vi "Dashboard Main.vi"() -> ()   [LabVIEW 2014]
uses:
  <vilib>/event_ctls.llb/eventvkey.ctl
  <vilib>/Rock Robotics/WPI/Dashboard/WPI_DashboardLogging Global.vi
  <vilib>/Utility/config.llb/Write Key (String).vi
  <vilib>/Utility/config.llb/Write Key (I32).vi
  <vilib>/Utility/config.llb/NI_LVConfig.lvlib
  Custom/BB_AutonomousSelector.lvlib
panel:
  in  "Rec Mode":enum32{"Stop", "Record", "Playback"}(radio)
  in  "Vision":u16(ring) items=["Camera Off", "USB Camera", "IP Camera"]
  out "Camera IP":string
  out "Image Message":string="Timeout in Camera Communications"
  in  "Dashboard Tab":T1(tab)
  in  "Autonomous\nMode":u16(ring) items=["Mars Rock", "BETA_1BALL_STRAIGHT", "BETA_1BALL_CENTER_R", "BETA_2BALL_CENTER_R", "BETA_2BALL_CENTER_L"]
  out "Battery":dbl(slide) scale=11.0..13.0
  in  "Camera Settings":T2={"Frame Rate"=30, "Compression"=30, "Size"=1} {"Frame Rate" scale=1.0..30.0; "Size" items=["640x480", "320x240", "160x120"]}
  out "Mode":T3(ring)=enum."Auto Disabled"
  in  "DB Camera Config":bool
  out "fps":dbl format="%#.1g"
  out "Mbps":dbl format="%#.1g"
  out "Mbps 2":bool
  out "Air Pressure":dbl(knob) scale=0.0..130.0
  in  "DB/String 9":string
  in  "DB/String 8":string
  in  "DB/String 7":string
  in  "DB/String 6":string
  in  "DB/String 5":string
  in  "DB/String 4":string
  in  "DB/String 3":string
  in  "DB/String 2":string
  in  "DB/String 1":string
  in  "DB/String 0":string
  in  "DB/Slider 0":dbl(slide) scale=0.0..5.0
  in  "DB/Slider 1":dbl(slide) scale=0.0..5.0
  in  "DB/Slider 2":dbl(slide) scale=0.0..5.0
  in  "DB/Slider 3":dbl(slide) scale=0.0..5.0
  out "DB/LED 3":bool
  out "DB/LED 2":bool
  out "DB/LED 1":bool
  out "DB/LED 0":bool
  in  "DB/Button 3":bool
  in  "DB/Button 2":bool
  in  "DB/Button 1":bool
  in  "DB/Button 0":bool
  in  "Test Slider":dbl(slide) scale=0.0..100.0 scale format="%#_3g"
  in  "On/Off":bool caption="Solenoid"
  in  "Test Name":u16(ring) items=["Select the test to run...", "Example Test", "-------------------------------", "List of tests is built in robot code.", "Replace with your own automated tests."]
  in  "Test Tree":string(tree)
  in  "Motor":cluster{"Value":dbl, "Enable":bool} {"Value" scale=-1.0..1.0 scale format="%#_3g"}
  out "Progress":T4 {"Test Progress" scale=0.0..100.0}
  in  "Rev/Fwd":cluster{"Forward":bool, "Reverse":bool}
  in  "Test Ring":u16(ring) items=["Auto", "Fixed indoor", "Fixed outdoor 1", "Fixed outdoor 2", "Fixed fluorescent 1", "Fixed fluorescent 2", "Hold current"]
  in  "Listbox":i32(listbox)
  out "Tree":string(tree)
  out "Camera Image":T5(plugin-control)
  out "Boolean":bool
  # "This tab is a great place for autonomous settings and robot-specific values.\nPlacie controls and indicators inside this tab and match name to\nDashboard Variables on robot. You can also delete this comment."
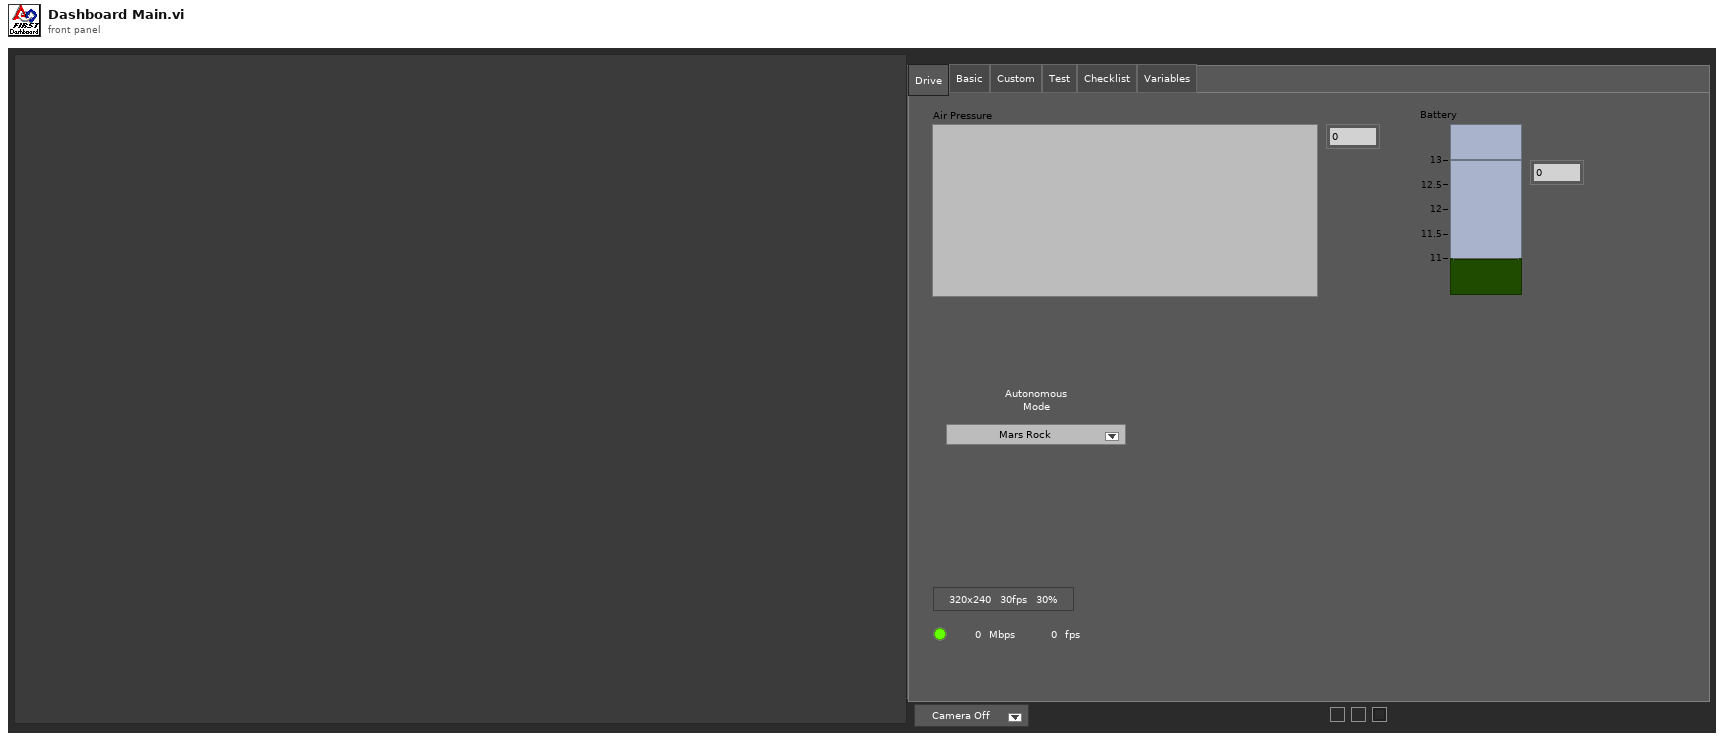
[diagram p1: front panel]
types:
  T1 = enum32{"Drive", "Basic", "Custom", "Test", "Checklist", "Variables"}
  T2 = cluster{"Frame Rate":i32, "Compression":i32, "Size":u16}
  T3 = enum8{"Tele-Op Disabled", "Tele-Op Enabled", "Auto Disabled", "Auto Enabled", "Test Disabled", "Test Enabled", ""}
  T4 = cluster{"Test Progress":u8, "Test Progress Text":string}
  T5 = typedef "IMAQ Image.ctl" = refnum<image>
  T6 = typedef "Image Type" = u32
  T7 = cluster{"Camera Image":refnum<vi>, "Dashboard Tab":refnum<vi>, "Boolean":refnum<vi>, "Vision":refnum<vi>, "Test Slider":refnum<vi>, "On/Off ":refnum<vi>, "Test Ring":refnum<vi>, "Rev/Fwd":refnum<vi>, "Rec Mode":refnum<vi>}
  T8 = cluster{"Digital Inputs":bool[], "Digital Outputs":bool[]}
  T9 = cluster{"Competition mode":bool, "Robot Link":bool, "Autonomous":bool, "Enabled":bool, "E-Stop":bool, "Simulated":bool, "TestMode":bool, "Docked Window":bool}
  T10 = typedef "NI_LVConfig.lvlib/Config Data RefNum.ctl" = refnum<k1>
  T11 = typedef "eventvkey.ctl" = enum16{"ASCII", "Enter", "Return", "Shift", "Ctrl", "Alt", "Cmd", "Opt", "Caps", "NumLock", "Clear", "Break", "Up", "Down", "Left", "Right", "Insert", "Delete", "Home", "End", "PageUp", "PageDown", "Escape", "Help", "Pause", "ScrollLock", "F1", "F2", "F3", "F4", "F5", "F6", "F7", "F8", "F9", "F10", "F11", "F12", "F13", "F14", "F15", "F16", "F17", "F18", "F19", "F20", "F21", "F22", "F23", "F24", "Play", "VolumeUp", "VolumeDown", "Mute", "Two Byte Char"}
  T12 = cluster{"Image Size":bool, "Image Type":bool, "Pixel Value":bool, "ROI Information":bool, "Zoom Factor":bool}
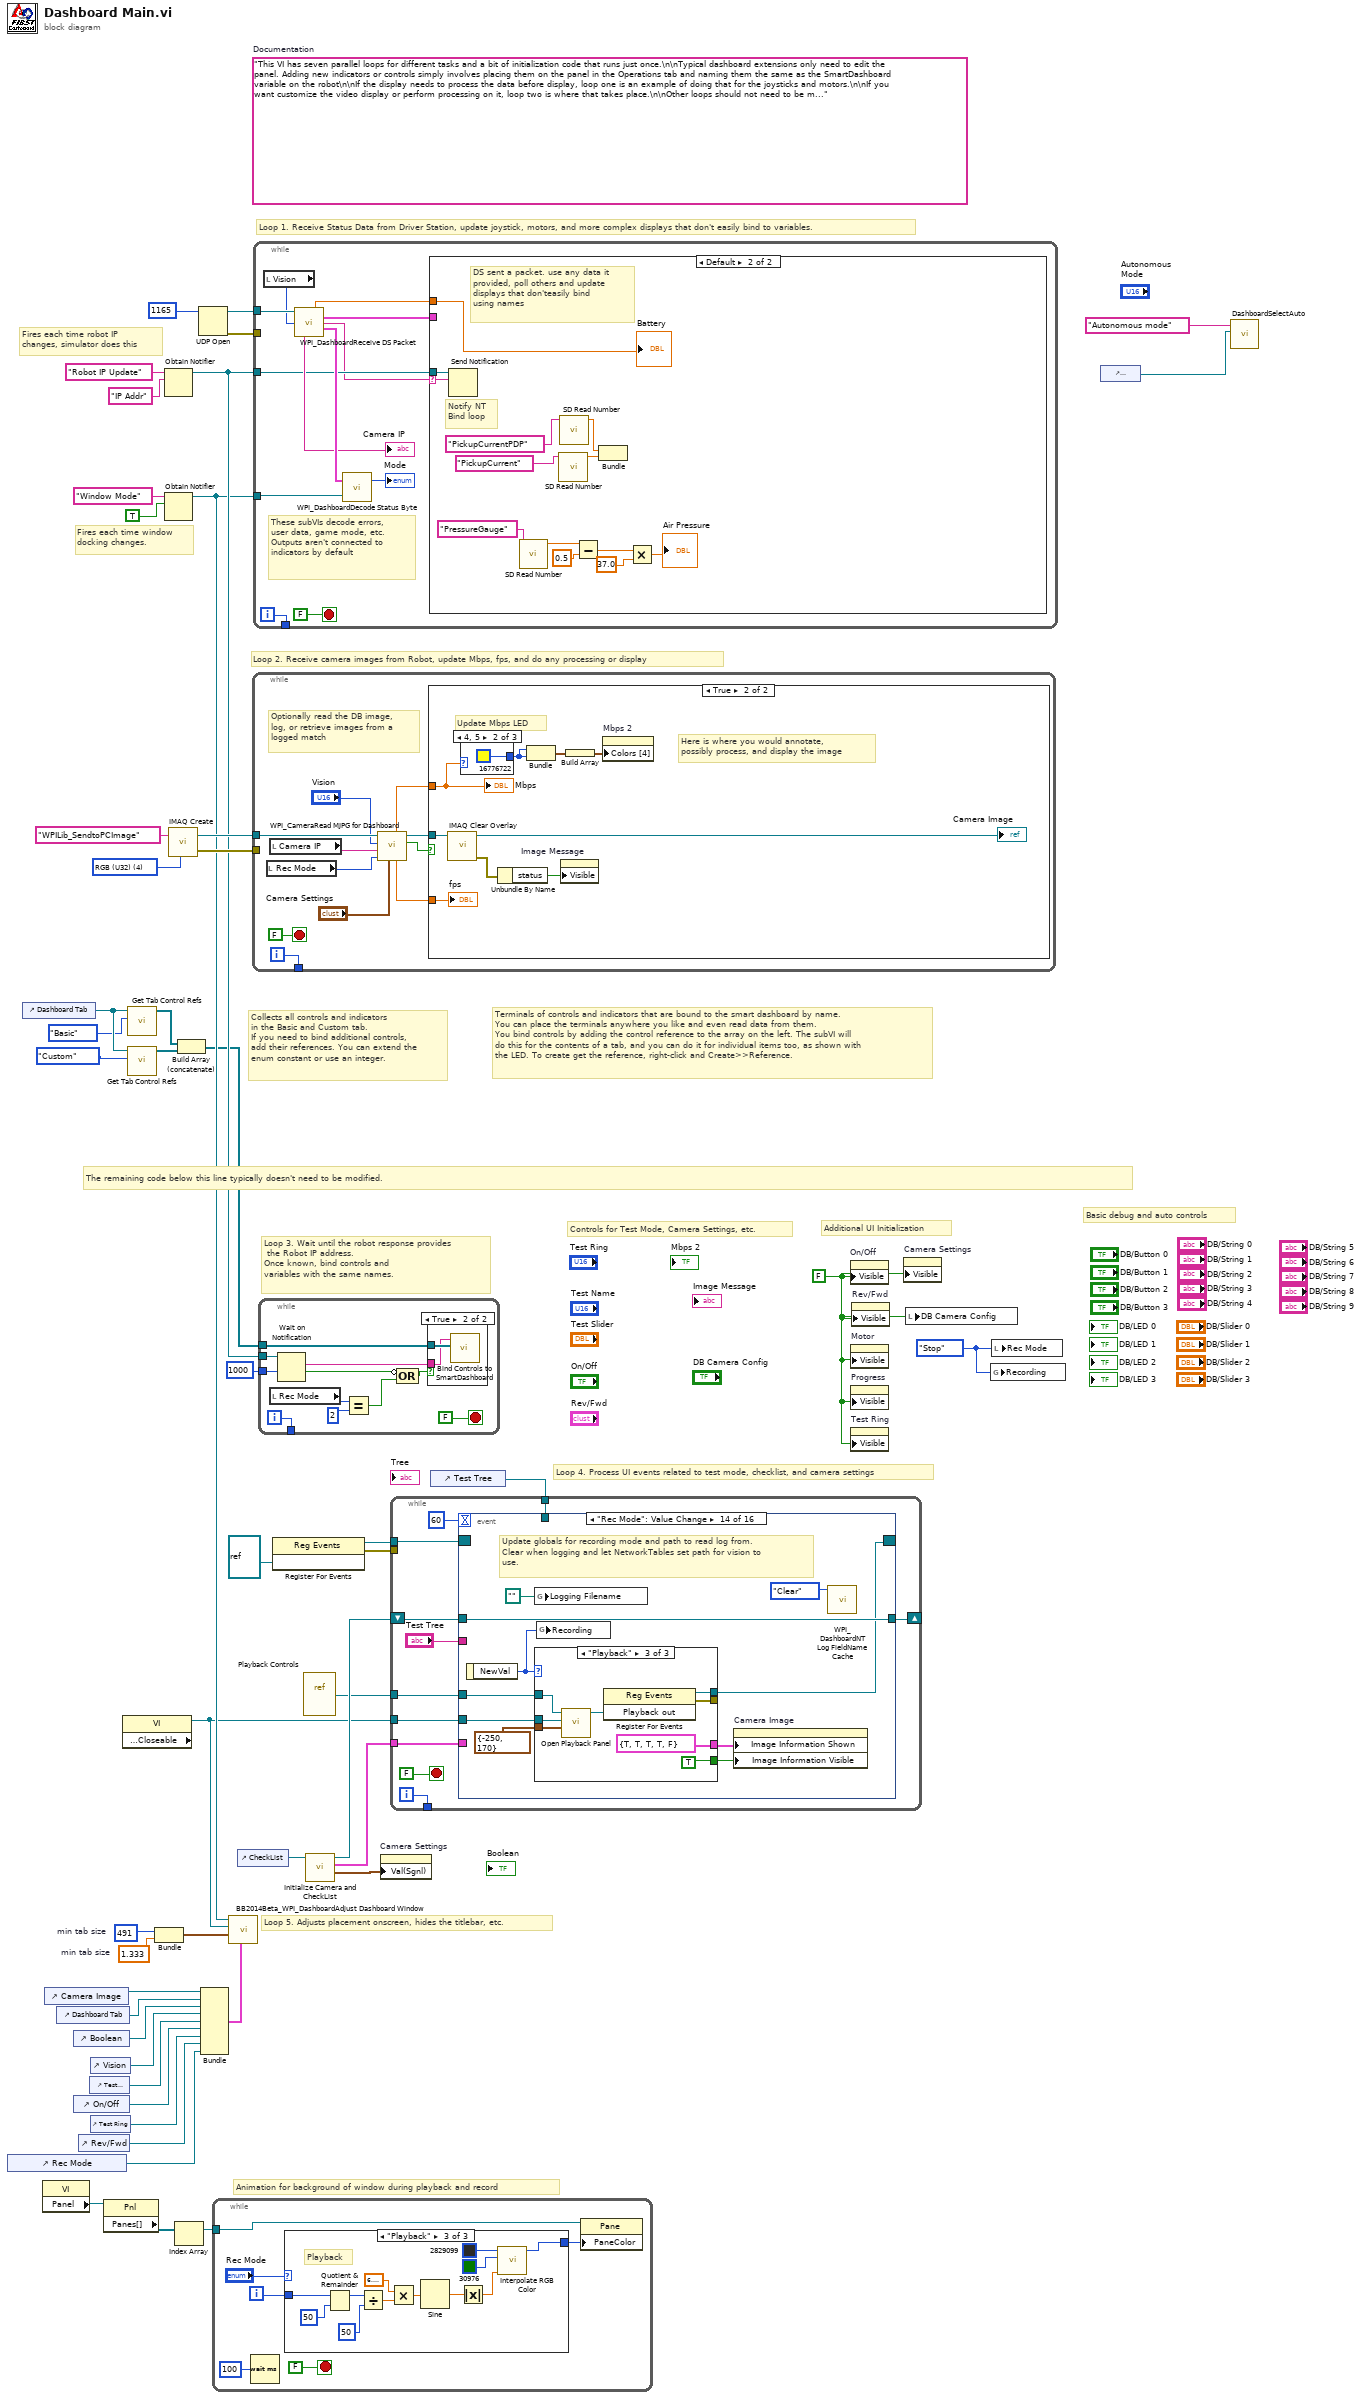
[diagram p0: block diagram]
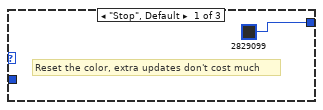
[diagram p2: hidden frame]
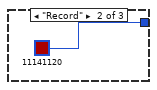
[diagram p3: hidden frame]
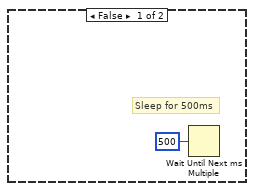
[diagram p5: hidden frame]
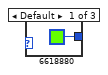
[diagram p6: hidden frame]
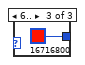
[diagram p7: hidden frame]
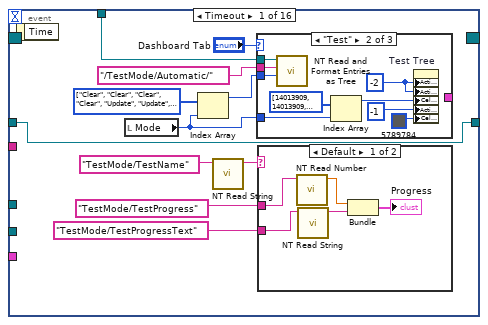
[diagram p8: hidden frame]
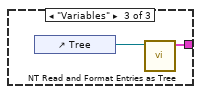
[diagram p10: hidden frame]
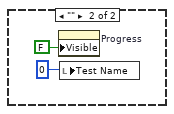
[diagram p11: hidden frame]
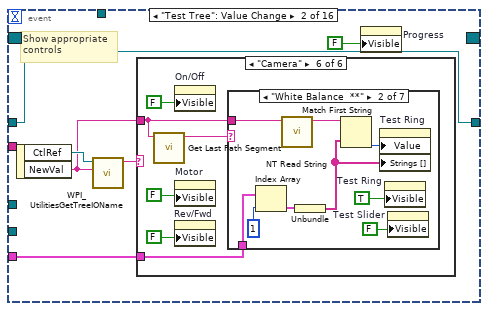
[diagram p12: hidden frame]
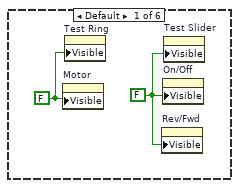
[diagram p13: hidden frame]
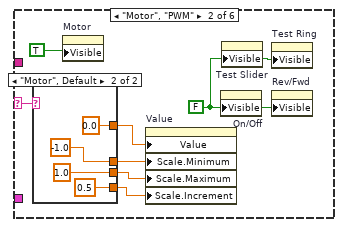
[diagram p14: hidden frame]
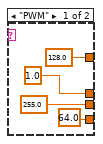
[diagram p15: hidden frame]
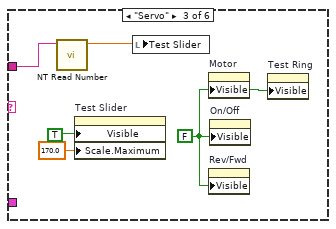
[diagram p16: hidden frame]
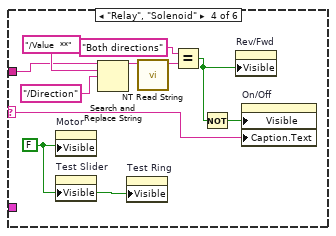
[diagram p17: hidden frame]
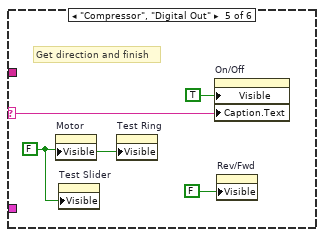
[diagram p18: hidden frame]
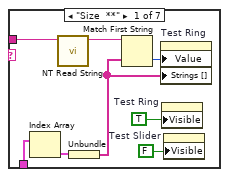
[diagram p19: hidden frame]
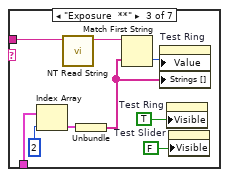
[diagram p20: hidden frame]
diagram:
  w10 = 491  # min tab size
  w9 = 1.333  # min tab size
  w24 = enum32{"Stop", "Record", "Playback"}."Stop" ("Rec Mode")
  w39 = FALSE ("Visible")
  (unwired) "This VI has seven parallel loops for different tasks and a bit of initialization code that runs just once.\n\nTypical dashboard extensions only need to edit the panel. Adding new indicators or controls simply involves placing them on the panel in the Operations tab and naming them the same as the SmartDashboard variable on the robot\n\nIf the display needs to process the data before display, loop one is an example of doing that for the joysticks and motors.\n\nIf you want customize the video display or perform processing on it, loop two is where that takes place.\n\nOther loops should not need to be modified. They are pretty standard, and document the task they perform."  # Documentation
  w48 = T6 4 items=["Grayscale (U8)", "Grayscale (I16)", "Grayscale (SGL)", "Complex (CSG)", "RGB (U32)", "HSL (U32)", "RGB (U64)"] ("Image Type")
  # "Basic debug and auto controls"
  # "Controls for Test Mode, Camera Settings, etc."
  # "Additional UI Initialization"
  # "Animation for background of window during playback and record"
  # "Fires each time robot IP\nchanges, simulator does this"
  # "Fires each time window\ndocking changes."
  # "Collects all controls and indicators\nin the Basic and Custom tab.\nIf you need to bind additional controls,\nadd their references. You can extend the\nenum constant or use an integer."
  # "The remaining code below this line typically doesn't need to be modified."
  # "Loop 4. Process UI events related to test mode, checklist, and camera settings"
  # "Terminals of controls and indicators that are bound to the smart dashboard by name.\nYou can place the terminals anywhere you like and even read data from them.\nYou bind controls by adding the control reference to the array on the left. The subVI will\ndo this for the contents of a tab, and you can do it for individual items too, as shown with\nthe LED. To create get the reference, right-click and Create>>Reference."
  # "Loop 3. Wait until the robot response provides\n the Robot IP address.\nOnce known, bind controls and\nvariables with the same names."
  # "Loop 5. Adjusts placement onscreen, hides the titlebar, etc."
  # "Loop 1. Receive Status Data from Driver Station, update joystick, motors, and more complex displays that don't easily bind to variables."
  # "Loop 2. Receive camera images from Robot, update Mbps, fps, and do any processing or display"
  n1 = control-ref of="Rec Mode"() -> (w11:refnum<vi>)
  n2 = control-ref of="Dashboard Tab"() -> (w22:refnum<vi>)
  n3 = property class="VI"() -> ("Panel"=w33:refnum<vi>)  [unwired: 2 in, 2 out]
  n4 = control-ref of="Camera Image"() -> (w18:refnum<vi>)
  n5 = control-ref of="Dashboard Tab"() -> (w17:refnum<vi>)
  n6 = control-ref of="Boolean"() -> (w7:refnum<vi>)
  n7 = control-ref of="On/Off"() -> (w14:refnum<vi>)
  n8 = control-ref of="Rev/Fwd"() -> (w12:refnum<vi>)
  n9 = control-ref of="Test Slider"() -> (w15:refnum<vi>)
  n10 = control-ref of="Vision"() -> (w16:refnum<vi>)
  n11 = control-ref of="Test Ring"() -> (w13:refnum<vi>)
  n12 = property class="Pnl"(reference=w33) -> ("Panes[]"=w34:refnum<vi>[])  [unwired: 1 in, 2 out]
  n13 = property class="VI" props=["Front Panel.Closeable"]() -> (reference out=w23:refnum<vi>)  [unwired: 2 in, 2 out]
  n14 = call <vilib>:"Get Tab Control Refs.vi"("Page Index"=T1."Basic" ("Dashboard Tab"), "TabControl in"=w22) -> ("ControlsOnPage"=w20:refnum<vi>[])  [unwired: 9 in]
  n15 = call <vilib>:"Get Tab Control Refs.vi"("Page Index"=T1."Custom" ("Dashboard Tab"), "TabControl in"=w22) -> ("ControlsOnPage"=w21:refnum<vi>[])  [unwired: 9 in]
  n16 = Bundle("min tab size"=w10, "min tab size"=w9) -> (w8:cluster{"min tab size":i32, "min tab size":dbl})  [unwired: 1 in]
  n17 = Obtain Notifier(name (unnamed)="Robot IP Update", notification data type="IP Addr" ("name (unnamed)")) -> (notifier out=w42:refnum<notifier>)  [unwired: 2 in, 2 out]
  n18 = Obtain Notifier(name (unnamed)="Window Mode", notification data type=TRUE) -> (notifier out=w26:refnum<notifier>)  [unwired: 2 in, 2 out]
  n19 = call "IMAQ Create"("Image Name"="WPILib_SendtoPCImage", "Image Type"=w48) -> ("New Image"=w46:T5, "error out"=w45:errorcluster)  [unwired: 2 in, 1 out]
  n20 = Index Array(array=w34) -> (element=w32:refnum<vi>)  [unwired: 1 in]
  n21 = Build Array (concatenate)(w20, w21) -> (w19:refnum<vi>[])
  n22 = UDP Open(11:u16 1165 ("port")) -> (port=w49:refnum<k16>, 0:w4:errorcluster)  [unwired: 2 in, 3 out]
  n23 = Bundle("Camera Image"=w18, "Dashboard Tab"=w17, "Boolean"=w7, "Vision"=w16, "Test Slider"=w15, "On/Off"=w14, "Test Ring"=w13, "Rev/Fwd"=w12, "Rec Mode"=w11) -> (w3:T7)  [unwired: 1 in]
  n24 = while {
    tunnel: w32 -> [w52]
    i -> [w55]
    stop <- FALSE stop-if-true
    n25 = Wait (ms)(milliseconds to wait=u32 100) -> ()  [unwired: 1 out]
    n26 = case shown="\"Playback\"" "Rec Mode" {
      tunnel: w55 -> [_ _ w70]
      tunnel: [u32 2829099 ("Base Color") u32 11141120 ("Target Color") w59] -> w51
      frame "Stop", Default {
        # "Reset the color, extra updates don't cost much"
      }
      frame "Record" {
      }
      frame "Playback" {
        # "Playback"
        n27 = Quotient & Remainder(x=w70, y=u32 50 ("milliseconds to wait")) -> (x-y*floor(x/y)=w66:u32)  [unwired: 1 out]
        n28 = Divide(x=w66, y=u32 50 ("milliseconds to wait")) -> (x/y=w63:dbl)
        n29 = Multiply(x=6.283185307179586, y=w63) -> (x*y=w68:dbl)
        n30 = Sine(x=w68) -> (sin(x)=w67:dbl)
        n31 = Absolute Value(x=w67) -> (abs(x)=w60:dbl)
        n32 = call "Interpolate RGB Color.vi"("Proportion"=w60, "Target Color"=u32 30976, "Base Color"=u32 2829099) -> ("Result Color"=w59:u32)  [unwired: 8 in]
      }
    }
    n33 = property class="Pane"(reference=w52, "PaneColor"=w51) -> ()  [unwired: 1 in, 2 out]
  }
  n34 = call "BB2014Beta_WPI_DashboardAdjust Dashboard Window.vi"("Sizing Refnums"=w3, "Size Constraints"=w8, "VI"=w23, "Notifier in"=w26) -> ()  [unwired: 8 in]
  n35 = control-ref of="CheckList"() -> (w25:refnum<vi>)
  n36 = while {
    tunnel: w46 -> [w79]
    tunnel: w45 -> [_]
    tunnel: [w80] -> _
    i -> [w80]
    stop <- FALSE stop-if-true
    # "Optionally read the DB image,\nlog, or retrieve images from a\nlogged match"
    n37 = local read "Rec Mode"() -> (w73:enum32{"Stop", "Record", "Playback"})
    n38 = local read "Camera IP"() -> (w71:string)
    n39 = call <vilib>:"WPI_CameraRead MJPG for Dashboard.vi"("Camera Settings"="Camera Settings", "Rec Mode"=w73, "Camera IP"=w71, "Vision"="Vision", "Refnum in"=w79) -> ("Active"=w77:bool, "Refnum out"=w78:T5, "FPS"=w76:dbl, "Bandwidth (Mbps)"=w75:dbl)  [unwired: 3 in]
    n40 = case shown="True" w77 {
      tunnel: w78 -> [_ w86]
      tunnel: w75 -> [_ w85]
      tunnel: w76 -> [_ w83]
      frame False {
        # "Sleep for 500ms"
        n41 = Wait Until Next ms Multiple(millisecond multiple=u32 500) -> ()  [unwired: 1 out]
      }
      frame True {
        # "Here is where you would annotate,\npossibly process, and display the image"
        # "Update Mbps LED"
        n42 = call "IMAQ Clear Overlay"("Image"=w86) -> ("error out"=w90:errorcluster, "Image Out"=→"Camera Image":T5)  [unwired: 2 in, 7 out]
        n43 = case shown="4, 5" w85 {
          tunnel: [u32 6618880 ("Color Box") u32 16776722 ("Color Box") u32 16716800 ("Color Box")] -> w87
          frame Default {
          }
          frame 4, 5 {
          }
          frame 6.. {
          }
        }
        n44 = Unbundle By Name(w90) -> ("status"=w91:bool)
        n45 = Bundle("Color Box"=w87, "Color Box"=w87) -> (w89:cluster{"Color Box":u32, "Color Box":u32})  [unwired: 1 out]
        n46 = property on="Image Message" class="Str"("Visible"=w91) -> ()  [unwired: 2 in, 2 out]
        n47 = Build Array(w89) -> (w88:cluster{"Color Box":u32, "Color Box":u32}[])
        n48 = property on="Mbps 2" class="Bool (strict)"("Colors [4]"=w88) -> ()  [unwired: 2 in, 2 out]
        "Mbps" <- w85
        "fps" <- w83
      }
    }
  }
  n49 = while {
    tunnel: w49 -> [w104]
    tunnel: w42 -> [w99]
    tunnel: w26 -> [w103]
    tunnel: [w100] -> _
    tunnel: w4 -> [_]
    i -> [w100]
    stop <- FALSE stop-if-true
    # "These subVIs decode errors, user data, game mode, etc.\nOutputs aren't connected to indicators by default"
    n50 = local read "Vision"() -> (w95:u16)
    n51 = call <vilib>:"WPI_DashboardReceive DS Packet.vi"("Recv Socket"=w104, "Vision"=w95) -> ("Battery"=w97:sgl, "Driver Station"=w98:T8, "Robot IP Address"=w96:string, "Status"=w105:T9, "Camera IP Address"=→"Camera IP":string)  [unwired: 1 in, 8 out]
    n52 = call <vilib>:"WPI_DashboardDecode Status Byte.vi"("Window Mode Notifier"=w103, "Status"=w105) -> ("Mode"=→"Mode":T3)  [unwired: 1 out]
    n53 = case shown="Default" w96 {
      selector: w96 -> [_ w118]
      tunnel: w99 -> [_ w119]
      tunnel: w98 -> [_ _]
      tunnel: w97 -> [_ w107]
      frame "0.0.0.0" {
        # "DS not sending packets, or no robot exists yet.\nDon't poll the variables"
      }
      frame Default {
        # "Notify NT\nBind loop"
        # "DS sent a packet. use any data it\nprovided, poll others and update\ndisplays that don'teasily bind\nusing names"
        n54 = Send Notification(notification=w118, notifier=w119) -> ()  [unwired: 1 in, 2 out]
        n55 = call <vilib>:"SD Read Number.vi"("Name"="PressureGauge") -> ("Numeric"=w116:dbl)  [unwired: 8 in, 2 out]
        n56 = call <vilib>:"SD Read Number.vi"("Name"="PickupCurrent") -> ("Numeric"=w110:dbl)  [unwired: 8 in, 2 out]
        n57 = call <vilib>:"SD Read Number.vi"("Name"="PickupCurrentPDP") -> ("Numeric"=w108:dbl)  [unwired: 8 in, 2 out]
        n58 = Subtract(x=w116, y=0.5) -> (x-y=w114:dbl)
        n59 = Bundle("Numeric"=w108, "Numeric"=w110) -> ()  [unwired: 1 in, 1 out]
        n60 = Multiply(x=w114, y=37.0) -> (x*y=→"Air Pressure":dbl)
        "Battery" <- w107
      }
    }
  }
  n61 = while {
    tunnel: w19 -> [w130]
    tunnel: w42 -> [w128]
    tunnel: [w126] -> _
    tunnel: u32 1000 ("milliseconds to wait") -> [w125]
    i -> [w126]
    stop <- FALSE stop-if-true
    n62 = local read "Rec Mode"() -> (w121:enum32{"Stop", "Record", "Playback"})
    n63 = Wait on Notification(notifier=w128, timeout in ms (-1)=w125) -> (notification=w127:string, timed out?=w123:bool)  [unwired: 2 in, 2 out]
    n64 = Equal?(x=w121, y=u16 2 ("Rec Mode")) -> (x = y?=w122:bool)
    n65 = Compound Arithmetic op=OR(invert w123, w122) -> (w124:bool)
    n66 = case shown="True" w124 {
      tunnel: w130 -> [_ w132]
      tunnel: w127 -> [_ w131]
      frame False {
      }
      frame True {
        n67 = call <vilib>:"Bind Controls to SmartDashboard.vi"("Bound Control Refs"=w132, "Server IP Address"=w131) -> ()  [unwired: 10 in]
      }
    }
  }
  n68 = register-events(refnum<vi> refnum) -> (reference out=w30:refnum<event-registration>, error out=w29:errorcluster)  [unwired: 2 in]
  n69 = vi-ref "Playback Controls.vi"() -> (w31:refnum<vi>)
  n70 = call "Initialize Camera and CheckList.vi"("ListBox in"=w25) -> ("Cluster"=w37:cluster{"value":i32, "value":i32, "index":i32}, "Array"=w38:cluster{string[]}[], "File Refnum"=w36:T10)  [unwired: 8 in]
  n71 = property on="Camera Settings" class="Clust (strict)"("Val(Sgnl)"=w37) -> ()  [unwired: 2 in, 2 out]
  n72 = control-ref of="Test Tree"() -> (w35:refnum<vi>)
  n73 = while {
    tunnel: w38 -> [w140]
    shift-right: [w139] -> _
    shift-left: w36 -> [w138]
    tunnel: [w137] -> _
    tunnel: w35 -> [w136]
    tunnel: w31 -> [w135]
    tunnel: w30 -> [w134]
    tunnel: w29 -> [_]
    tunnel: w23 -> [w133]
    i -> [w137]
    stop <- FALSE stop-if-true
    n74 = event shown="[13] \"Rec Mode\": Value Change" {
      selector: w134 -> [_ _ _ _ _ _ _ _ _ _ _ _ _ _ _ _]
      dyn-events: [_ _ _ _ _ _ _ _ _ _ _ _ _ w378 _ _] -> _
      timeout: u32 60 ("milliseconds to wait") -> [_ _ _ _ _ _ _ _ _ _ _ _ _ _ _ _]
      tunnel: w136 -> [w150 _ _ _ _ _ _ _ _ _ _ _ _ _ _ _]
      tunnel: "Test Tree" -> [_ _ _ _ _ _ _ _ w347 w355 w357 w361 w369 _ _ _]
      tunnel: w140 -> [_ w174 _ _ _ _ w311 w341 _ _ _ _ _ _ _ _]
      tunnel: [w144 w173 w272 w277 w285 w297 w310 w334 w346 w353 w356 w360 w368 w380 w394 w395] -> w139
      tunnel: w138 -> [w144 w173 w272 w277 w285 w297 w309 w334 w346 w353 w356 w360 w368 w380 w394 w395]
      tunnel: w135 -> [_ _ _ _ _ _ _ _ _ _ _ _ _ w381 _ w398]
      tunnel: w133 -> [_ _ _ _ _ _ _ _ _ _ _ _ _ w376 _ _]
      event Timeout {
        w149 = enum16{"Update", "Clear"}[] [enum."Clear", enum."Clear", enum."Clear", enum."Clear", enum."Update", enum."Update", enum."Clear"] items=["Update", "Clear"]
        n75 = event-data() -> ()  [unwired: 1 in, 1 out]
        n76 = local read "Mode"() -> (w147:T3)
        n77 = Index Array(array=w149, index=w147) -> (element=w148:enum16{"Update", "Clear"})
        n78 = call <vilib>:"NT Read String.vi"("Name"="TestMode/TestName") -> ("String"=w153:string)  [unwired: 9 in, 1 out]
        n79 = case shown="\"Test\"" "Dashboard Tab" {
          tunnel: w150 -> [_ w163 _]
          tunnel: "/TestMode/Automatic/" ("Name Pattern") -> [_ w162 _]
          tunnel: w148 -> [_ w161 _]
          tunnel: w147 -> [_ w159 _]
          tunnel: [_ _ w165] -> _
          frame "Custom", Default {
          }
          frame "Test" {
            w158 = -2 ("Active Item:Row Number")
            n80 = call <vilib>:"NT Read and Format Entries as Tree.vi"("Operation"=w161, "Name Pattern"=w162, "Tree Refnum"=w163) -> ()  [unwired: 7 in, 2 out]
            n81 = Index Array(array=u32[] [14013909, 14013909, 14013909, 14013909, 14013909, 16777215, 14013909], index=w159) -> (element=w157:u32)
            n82 = property on="Test Tree" class="Tree (strict)"("Active Item Row Number"=w158, "ActiveColNum"=w158, "CellBG"=w157, "Active Item Row Number"=-1 ("Active Item:Row Number"), "CellBG"=u32 5789784 ("Color Box")) -> ()  [unwired: 2 in, 2 out]
          }
          frame "Variables" {
            n83 = control-ref of="Tree"() -> (w164:refnum<vi>)
            n84 = call <vilib>:"NT Read and Format Entries as Tree.vi"("Tree Refnum"=w164) -> ("Formatted Strings"=w165:cluster{"Name":string, "Value":string}[])  [unwired: 9 in, 1 out]
          }
        }
        n85 = case shown="Default" w153 {
          tunnel: "TestMode/TestProgress" ("Name") -> [w167 _]
          tunnel: "TestMode/TestProgressText" ("Name") -> [w166 _]
          frame Default {
            n86 = call <vilib>:"NT Read Number.vi"("Name"=w167) -> ("Numeric"=w168:dbl)  [unwired: 9 in, 1 out]
            n87 = call <vilib>:"NT Read String.vi"("Name"=w166) -> ("String"=w169:string)  [unwired: 9 in, 1 out]
            n88 = Bundle("Numeric"=w168, "String"=w169) -> (→"Progress":cluster{"Numeric":dbl, "String":string})  [unwired: 1 in]
          }
          frame "" {
            n89 = property on="Progress" class="Clust (strict)"("Visible"=FALSE) -> ()  [unwired: 2 in, 2 out]
            n90 = local write "Test Name"(u16 0) -> ()
          }
        }
      }
      event "Test Tree": Value Change {
        # "Show appropriate\ncontrols"
        n91 = event-data() -> ("CtlRef"=w177:refnum<vi>, "NewVal"=w175:string)  [unwired: 1 in]
        n92 = call <vilib>:"WPI_UtilitiesGetTreeIOName.vi"("NewVal"=w175, "TreeControl in"=w177) -> ("I/O Name"=w178:string)  [unwired: 9 in]
        n93 = case shown="\"Camera\"" w178 {
          selector: w178 -> [_ w185 _ w203 w212 _]
          tunnel: w175 -> [_ _ w200 w202 _ w219]
          tunnel: w174 -> [_ _ _ _ _ w218]
          frame Default {
            w180 = FALSE ("Visible")
            w179 = FALSE ("Visible")
            n94 = property on="Motor" class="Clust (strict)"("Visible"=w179) -> ()  [unwired: 2 in, 2 out]
            n95 = property on="Test Ring" class="Ring (strict)"("Visible"=w179) -> ()  [unwired: 2 in, 2 out]
            n96 = property on="Rev/Fwd" class="Clust (strict)"("Visible"=w180) -> ()  [unwired: 2 in, 2 out]
            n97 = property on="On/Off" class="Bool (strict)"("Visible"=w180) -> ()  [unwired: 2 in, 2 out]
            n98 = property on="Test Slider" class="Slide (strict)"("Visible"=w180) -> ()  [unwired: 2 in, 2 out]
          }
          frame "Motor", "PWM" {
            w186 = FALSE ("Visible")
            n99 = case shown="\"Motor\", Default" w185 {
              tunnel: [1.0 ("Value") -1.0 ("Value")] -> w184
              tunnel: [255.0 ("Value") 1.0 ("Value")] -> w183
              tunnel: [128.0 ("Value") 0.0 ("Value")] -> w182
              tunnel: [64.0 ("Value") 0.5 ("Value")] -> w181
              frame "PWM" {
              }
              frame "Motor", Default {
              }
            }
            n100 = property on="Motor" class="Clust (strict)"("Visible"=TRUE) -> ()  [unwired: 2 in, 2 out]
            n101 = property on="Value" class="Slide (strict)"("Value"=w182, "Scale.Minimum"=w184, "Scale.Maximum"=w183, "Scale.Increment"=w181) -> ()  [unwired: 2 in, 2 out]
            n102 = property on="On/Off" class="Bool (strict)"("Visible"=w186) -> ()  [unwired: 2 in, 2 out]
            n103 = property on="Test Slider" class="Slide (strict)"("Visible"=w186) -> ()  [unwired: 2 in, 2 out]
            n104 = property on="Test Ring" class="Ring (strict)"("Visible"=w186) -> ()  [unwired: 2 in, 2 out]
            n105 = property on="Rev/Fwd" class="Clust (strict)"("Visible"=w186) -> ()  [unwired: 2 in, 2 out]
          }
          frame "Servo" {
            w198 = FALSE ("Visible")
            n106 = call <vilib>:"NT Read Number.vi"("Name"=w200) -> ("Numeric"=w199:dbl)  [unwired: 9 in, 1 out]
            n107 = property on="Test Slider" class="Slide (strict)"("Visible"=TRUE, "Scale.Maximum"=170.0 ("Scale.Range:Maximum")) -> ()  [unwired: 2 in, 2 out]
            n108 = local write "Test Slider"(w199) -> ()
            n109 = property on="Motor" class="Clust (strict)"("Visible"=w198) -> ()  [unwired: 2 in, 2 out]
            n110 = property on="Rev/Fwd" class="Clust (strict)"("Visible"=w198) -> ()  [unwired: 2 in, 2 out]
            n111 = property on="On/Off" class="Bool (strict)"("Visible"=w198) -> ()  [unwired: 2 in, 2 out]
            n112 = property on="Test Ring" class="Ring (strict)"("Visible"=w198) -> ()  [unwired: 2 in, 2 out]
          }
          frame "Relay", "Solenoid" {
            w201 = FALSE ("Visible")
            n113 = property on="Motor" class="Clust (strict)"("Visible"=w201) -> ()  [unwired: 2 in, 2 out]
            n114 = property on="Test Slider" class="Slide (strict)"("Visible"=w201) -> ()  [unwired: 2 in, 2 out]
            n115 = Search and Replace String(input string=w202, search string="/Value  **", replace string="/Direction") -> (result string=w208:string)  [unwired: 5 in, 3 out]
            n116 = property on="Test Ring" class="Ring (strict)"("Visible"=w201) -> ()  [unwired: 2 in, 2 out]
            n117 = call <vilib>:"NT Read String.vi"("Name"=w208) -> ("String"=w206:string)  [unwired: 9 in, 1 out]
            n118 = Equal?(x="Both directions", y=w206) -> (x = y?=w204:bool)
            n119 = Not(x=w204) -> (.not. x?=w205:bool)
            n120 = property on="Rev/Fwd" class="Clust (strict)"("Visible"=w204) -> ()  [unwired: 2 in, 2 out]
            n121 = property on="On/Off" class="Bool (strict)"("Visible"=w205, "Caption.Text"=w203) -> ()  [unwired: 2 in, 2 out]
          }
          frame "Compressor", "Digital Out" {
            w211 = FALSE ("Visible")
            # "Get direction and finish"
            n122 = property on="Motor" class="Clust (strict)"("Visible"=w211) -> ()  [unwired: 2 in, 2 out]
            n123 = property on="Test Slider" class="Slide (strict)"("Visible"=w211) -> ()  [unwired: 2 in, 2 out]
            n124 = property on="Test Ring" class="Ring (strict)"("Visible"=w211) -> ()  [unwired: 2 in, 2 out]
            n125 = property on="On/Off" class="Bool (strict)"("Visible"=TRUE, "Caption.Text"=w212) -> ()  [unwired: 2 in, 2 out]
            n126 = property on="Rev/Fwd" class="Clust (strict)"("Visible"=FALSE) -> ()  [unwired: 2 in, 2 out]
          }
          frame "Camera" {
            n127 = call <vilib>:"Get Last Path Segment.vi"("String in"=w219) -> ("String out"=w220:string)  [unwired: 10 in]
            n128 = property on="On/Off" class="Bool (strict)"("Visible"=FALSE) -> ()  [unwired: 2 in, 2 out]
            n129 = property on="Motor" class="Clust (strict)"("Visible"=FALSE) -> ()  [unwired: 2 in, 2 out]
            n130 = property on="Rev/Fwd" class="Clust (strict)"("Visible"=FALSE) -> ()  [unwired: 2 in, 2 out]
            n131 = case shown="\"White Balance  **\"" w220 {
              tunnel: w219 -> [w226 w235 w244 w253 w262 _ w268]
              tunnel: w218 -> [w224 w232 w241 w250 w259 _ _]
              frame "Size  **" {
                n132 = Index Array(array=w224) -> (element=w223:cluster{string[]})  [unwired: 1 in]
                n133 = call <vilib>:"NT Read String.vi"("Name"=w226) -> ("String"=w225:string)  [unwired: 9 in, 1 out]
                n134 = Unbundle(w223) -> (w221:string[])
                n135 = Match First String(2:w221, 3:w225) -> (0:w222:i32)  [unwired: 1 out]
                n136 = property on="Test Ring" class="Ring (strict)"("Value"=w222, "Strings []"=w221) -> ()  [unwired: 2 in, 2 out]
                n137 = property on="Test Ring" class="Ring (strict)"("Visible"=TRUE) -> ()  [unwired: 2 in, 2 out]
                n138 = property on="Test Slider" class="Slide (strict)"("Visible"=FALSE) -> ()  [unwired: 2 in, 2 out]
              }
              frame "White Balance  **" {
                n139 = Index Array(array=w232, index=1) -> (element=w233:cluster{string[]})
                n140 = call <vilib>:"NT Read String.vi"("Name"=w235) -> ("String"=w234:string)  [unwired: 9 in, 1 out]
                n141 = Unbundle(w233) -> (w230:string[])
                n142 = Match First String(2:w230, 3:w234) -> (0:w229:i32)  [unwired: 1 out]
                n143 = property on="Test Ring" class="Ring (strict)"("Value"=w229, "Strings []"=w230) -> ()  [unwired: 2 in, 2 out]
                n144 = property on="Test Ring" class="Ring (strict)"("Visible"=TRUE) -> ()  [unwired: 2 in, 2 out]
                n145 = property on="Test Slider" class="Slide (strict)"("Visible"=FALSE) -> ()  [unwired: 2 in, 2 out]
              }
              frame "Exposure  **" {
                n146 = Index Array(array=w241, index=2) -> (element=w242:cluster{string[]})
                n147 = call <vilib>:"NT Read String.vi"("Name"=w244) -> ("String"=w243:string)  [unwired: 9 in, 1 out]
                n148 = Unbundle(w242) -> (w238:string[])
                n149 = Match First String(2:w238, 3:w243) -> (0:w239:i32)  [unwired: 1 out]
                n150 = property on="Test Ring" class="Ring (strict)"("Value"=w239, "Strings []"=w238) -> ()  [unwired: 2 in, 2 out]
                n151 = property on="Test Ring" class="Ring (strict)"("Visible"=TRUE) -> ()  [unwired: 2 in, 2 out]
                n152 = property on="Test Slider" class="Slide (strict)"("Visible"=FALSE) -> ()  [unwired: 2 in, 2 out]
              }
              frame "Exposure Priority  **" {
                n153 = Index Array(array=w250, index=3) -> (element=w251:cluster{string[]})
                n154 = call <vilib>:"NT Read String.vi"("Name"=w253) -> ("String"=w252:string)  [unwired: 9 in, 1 out]
                n155 = Unbundle(w251) -> (w247:string[])
                n156 = Match First String(2:w247, 3:w252) -> (0:w248:i32)  [unwired: 1 out]
                n157 = property on="Test Ring" class="Ring (strict)"("Value"=w248, "Strings []"=w247) -> ()  [unwired: 2 in, 2 out]
                n158 = property on="Test Ring" class="Ring (strict)"("Visible"=TRUE) -> ()  [unwired: 2 in, 2 out]
                n159 = property on="Test Slider" class="Slide (strict)"("Visible"=FALSE) -> ()  [unwired: 2 in, 2 out]
              }
              frame "Color Enable  **" {
                n160 = Index Array(array=w259, index=4) -> (element=w260:cluster{string[]})
                n161 = call <vilib>:"NT Read String.vi"("Name"=w262) -> ("String"=w261:string)  [unwired: 9 in, 1 out]
                n162 = Unbundle(w260) -> (w256:string[])
                n163 = Match First String(2:w256, 3:w261) -> (0:w257:i32)  [unwired: 1 out]
                n164 = property on="Test Ring" class="Ring (strict)"("Value"=w257, "Strings []"=w256) -> ()  [unwired: 2 in, 2 out]
                n165 = property on="Test Ring" class="Ring (strict)"("Visible"=TRUE) -> ()  [unwired: 2 in, 2 out]
                n166 = property on="Test Slider" class="Slide (strict)"("Visible"=FALSE) -> ()  [unwired: 2 in, 2 out]
              }
              frame Default {
                n167 = property on="Test Ring" class="Ring (strict)"("Visible"=FALSE) -> ()  [unwired: 2 in, 2 out]
                n168 = property on="Test Slider" class="Slide (strict)"("Visible"=FALSE) -> ()  [unwired: 2 in, 2 out]
              }
              frame "Brightness  **", "Color Level  **", "Compression  **", "FPS  **", "Sharpness  **" {
                n169 = call <vilib>:"NT Read Number.vi"("Name"=w268) -> ("Numeric"=w267:dbl)  [unwired: 9 in, 1 out]
                n170 = local write "Test Slider"(w267) -> ()
                n171 = property on="Test Slider" class="Slide (strict)"("Visible"=TRUE, "Scale.Maximum"=100.0 ("Scale.Range:Maximum")) -> ()  [unwired: 2 in, 2 out]
                n172 = property on="Test Ring" class="Ring (strict)"("Visible"=FALSE) -> ()  [unwired: 2 in, 2 out]
              }
            }
          }
        }
        n173 = property on="Progress" class="Clust (strict)"("Visible"=FALSE) -> ()  [unwired: 2 in, 2 out]
      }
      event "Test Name": Mouse Enter {
        # "Populate the ring with the list of tests"
        n174 = event-data() -> ()  [unwired: 1 in, 1 out]
        n175 = call <vilib>:"NT Read String Array.vi"("Name"="TestMode/TestList") -> ("String Array"=w276:string[])  [unwired: 9 in, 1 out]
        n176 = Build Array (concatenate)("Select the test to run...", w276) -> (w275:string[])
        n177 = property on="Test Name" class="Ring (strict)"("Strings []"=w275) -> ()  [unwired: 2 in, 2 out]
      }
      event "Test Name": Value Change {
        w278 = FALSE ("Visible")
        # "Tell the robot the test name to run"
        n178 = event-data() -> ("NewVal"=w282:u16)  [unwired: 1 in]
        n179 = property on="Test Name" class="Ring (strict)"() -> ("Strings []"=w283:string[])  [unwired: 2 in, 2 out]
        n180 = local write "Progress"(T4 {"Test Progress"=0, "Test Progress Text"=""} ("Progress")) -> ()
        n181 = Index Array(array=w283, index=w282) -> (element=w281:string)
        n182 = call <vilib>:"NT Write String.vi"("String"=w281, "Name"="TestMode/TestName") -> ()  [unwired: 9 in, 1 out]
        n183 = property on="Progress" class="Clust (strict)"("Visible"=TRUE) -> ()  [unwired: 2 in, 2 out]
        n184 = property on="Motor" class="Clust (strict)"("Visible"=w278) -> ()  [unwired: 2 in, 2 out]
        n185 = property on="Test Slider" class="Slide (strict)"("Visible"=w278) -> ()  [unwired: 2 in, 2 out]
        n186 = property on="On/Off" class="Bool (strict)"("Visible"=w278) -> ()  [unwired: 2 in, 2 out]
        n187 = property on="Rev/Fwd" class="Clust (strict)"("Visible"=w278) -> ()  [unwired: 2 in, 2 out]
        n188 = property on="Test Ring" class="Ring (strict)"("Visible"=w278) -> ()  [unwired: 2 in, 2 out]
      }
      event "Listbox": Double Click {
        n189 = event-data() -> ("PlatMods.Shift"=w286:bool, "Row"=w288:i32)  [unwired: 1 in]
        n190 = case shown="True" w286 {
          tunnel: w288 -> [w292 _]
          tunnel: 1 -> [w291 _]
          frame False {
            n191 = property on="Listbox" class="LstBox (strict)"() -> ("Item Symbols"=w290:i32[])  [unwired: 2 in, 2 out]
            n192 = Replace Array Subset(array=w290, new element=w291, index=w292) -> (w289:i32[])
            n193 = property on="Listbox" class="LstBox (strict)"("Item Symbols"=w289) -> ()  [unwired: 2 in, 2 out]
          }
          frame True {
            w293 = 0 ("Top Row")
            n194 = property on="Listbox" class="LstBox (strict)"() -> ("Number of Rows"=w295:u32)  [unwired: 2 in, 2 out]
            n195 = Initialize Array(0, w295) -> (w294:i32[])
            n196 = property on="Listbox" class="LstBox (strict)"("Top Row"=w293, "Value"=w293, "Item Symbols"=w294) -> ()  [unwired: 2 in, 2 out]
          }
        }
      }
      event "Listbox": Key Down {
        n197 = event-data() -> ("VKey"=w299:T11)  [unwired: 1 in]
        n198 = case shown="\"Left\", \"Right\"" w299 {
          selector: w299 -> [w304 _]
          tunnel: eventvkey."Left" ("VKey") -> [w302 _]
          frame "Left", "Right" {
            n199 = Equal?(x=w302, y=w304) -> (x = y?=w303:bool)
            n200 = Select(t=0, s=w303, f=1) -> (s? t:f=w305:i32)
            n201 = property on="Listbox" class="LstBox (strict)"() -> ("Item Symbols"=w308:i32[])  [unwired: 2 in, 2 out]
            n202 = Replace Array Subset(array=w308, new element=w305, index="Listbox") -> (w307:i32[])
            n203 = property on="Listbox" class="LstBox (strict)"("Item Symbols"=w307) -> ()  [unwired: 2 in, 2 out]
          }
          frame Default {
          }
        }
      }
      event "DB Camera Config": Value Change {
        n204 = event-data() -> ("NewVal"=w312:bool)  [unwired: 1 in]
        n205 = case shown="True" w312 {
          tunnel: w311 -> [w321 _]
          tunnel: [w314 w332] -> w310
          tunnel: w309 -> [w313 w332]
          frame False {
            w328 = "Camera"
            w331 = FALSE ("Visible")
            n206 = local read "Camera Settings"() -> (w320:T2)
            n207 = Index Array(array=w321) -> (element=w324:cluster{string[]})  [unwired: 1 in]
            n208 = Unbundle(w320) -> ("Frame Rate"=w319:i32, "Compression"=w318:i32, "Size"=w322:u16)
            n209 = Unbundle(w324) -> (w323:string[])
            n210 = Index Array(array=w323, index=w322) -> (element=w317:string)
            n211 = call-poly <vilib>:"Write Key.vi"("section"=w328, "value"=w317, "key"="Size", "refnum"=w313) -> ("refnum out"=w330:T10)  [unwired: 2 in, 5 out]
            n212 = call-poly <vilib>:"Write Key.vi"("section"=w328, "value"=w319, "key"="FrameRate", "refnum"=w330) -> ("refnum out"=w329:T10)  [unwired: 1 in, 6 out]
            n213 = property on="Camera Settings" class="Clust (strict)"("Visible"=w331) -> ()  [unwired: 2 in, 2 out]
            n214 = local write "DB Camera Config"(w331) -> ()
            n215 = call-poly <vilib>:"Write Key.vi"("section"=w328, "value"=w318, "key"="Compression", "refnum"=w329) -> ("refnum out"=w315:T10)  [unwired: 1 in, 6 out]
            n216 = call <vilib>:"Close Config Data.vi"("refnum"=w315) -> ("file path"=w316:path)  [unwired: 2 in, 8 out]
            n217 = call <vilib>:"Open Config Data.vi"("configuration file path"=w316) -> ("refnum"=w314:T10)  [unwired: 8 in, 2 out]
          }
          frame True {
            n218 = property on="Camera Settings" class="Clust (strict)"("Visible"=TRUE) -> ()  [unwired: 2 in, 2 out]
          }
        }
      }
      event "Camera Settings": Value Change {
        n219 = event-data() -> ("NewVal"=w345:T2)  [unwired: 1 in]
        n220 = Index Array(array=w341) -> (element=w340:cluster{string[]})  [unwired: 1 in]
        n221 = Unbundle(w345) -> ("Frame Rate"=w336:i32, "Compression"=w335:i32, "Size"=w338:u16)
        n222 = Unbundle(w340) -> (w339:string[])
        n223 = Index Array(array=w339, index=w338) -> (element=w337:string)
        n224 = Format Into String(format string="%s   %dfps   %d%%", w337, w336, w335) -> (resulting string=w342:string)  [unwired: 2 in, 1 out]
        n225 = Build Array(w342) -> (w343:string[])
        n226 = property on="DB Camera Config" class="Bool (strict)"("Strings [4]"=w343) -> ()  [unwired: 2 in, 2 out]
      }
      event "Motor.Enable": Value Change {
        n227 = event-data() -> ("NewVal"=w351:bool)  [unwired: 1 in]
        n228 = Unbundle("Motor") -> ("Value"=w350:dbl)  [unwired: 1 out]
        n229 = Select(t=w350, s=w351, f=0.0) -> (s? t:f=w348:dbl)
        n230 = call <vilib>:"NT Write Number.vi"("Numeric"=w348, "Name"=w347) -> ()  [unwired: 9 in, 1 out]
      }
      event "Test Slider": Value Change {
        n231 = event-data() -> ("NewVal"=w354:dbl)  [unwired: 1 in]
        n232 = call <vilib>:"NT Write Number.vi"("Numeric"=w354, "Name"=w355) -> ()  [unwired: 9 in, 1 out]
      }
      event "On/Off": Value Change {
        n233 = event-data() -> ("NewVal"=w359:bool)  [unwired: 1 in]
        n234 = Boolean To (0,1)(Boolean=w359) -> (0, 1=w358:i16)
        n235 = call <vilib>:"NT Write Number.vi"("Numeric"=w358, "Name"=w357) -> ()  [unwired: 9 in, 1 out]
      }
      event "Rev/Fwd": Value Change {
        n236 = event-data() -> ("NewVal.Forward"=w367:bool, "NewVal.Reverse"=w366:bool)  [unwired: 1 in]
        n237 = Boolean To (0,1)(Boolean=w367) -> (0, 1=w363:i16)
        n238 = Boolean To (0,1)(Boolean=w366) -> (0, 1=w365:i16)
        n239 = Negate(x=w365) -> (-x=w364:i16)
        n240 = Add(x=w363, y=w364) -> (x+y=w362:i16)
        n241 = call <vilib>:"NT Write Number.vi"("Numeric"=w362, "Name"=w361) -> ()  [unwired: 9 in, 1 out]
      }
      event "Test Ring": Value Change {
        n242 = event-data() -> ("NewVal"=w371:u16)  [unwired: 1 in]
        n243 = property on="Test Ring" class="Ring (strict)"() -> ("Strings []"=w372:string[])  [unwired: 2 in, 2 out]
        n244 = Index Array(array=w372, index=w371) -> (element=w370:string)
        n245 = call <vilib>:"NT Write String.vi"("String"=w370, "Name"=w369) -> ()  [unwired: 9 in, 1 out]
      }
      event "Rec Mode": Value Change {
        # "Update globals for recording mode and path to read log from.\nClear when logging and let NetworkTables set path for vision to\nuse."
        n246 = event-data() -> ("NewVal"=w382:enum32{"Stop", "Record", "Playback"})  [unwired: 1 in]
        n247 = global write "WPI_DashboardLogging Global.vi" "Logging Filename"(path "") -> ()
        n248 = case shown="\"Playback\"" w382 {
          tunnel: w381 -> [_ w384 w392]
          tunnel: [_ _ w391] -> w378
          tunnel: [_ _ w390] -> _
          tunnel: w376 -> [_ _ w388]
          tunnel: cluster{i32, i32} {-250, 170} -> [_ _ w387]
          tunnel: [_ _ T12 {"Image Size"=TRUE, "Image Type"=TRUE, "Pixel Value"=TRUE, "ROI Information"=TRUE, "Zoom Factor"=FALSE} ("Image Information Shown:All Elements")] -> w374
          tunnel: [_ _ TRUE ("Zoom Factor")] -> w373
          frame Default {
          }
          frame "Stop", "Record" {
            # "Place Window too"
            n249 = invoke class="VI" method="FP.Close"(reference=w384) -> (reference out=w383:refnum<vi>)  [unwired: 2 in, 2 out]
            n250 = invoke class="VI" method="Abort VI"(reference=w383) -> ()  [unwired: 2 in, 3 out]
          }
          frame "Playback" {
            n251 = call "Open Playback Panel.vi"("Offset"=w387, "DB VI Ref"=w388, "Playback in"=w392) -> ("Playback out"=w389:refnum<vi>)  [unwired: 8 in]
            n252 = register-events(w389) -> (reference out=w391:refnum<event-registration>, error out=w390:errorcluster)  [unwired: 2 in]
          }
        }
        n253 = global write "WPI_DashboardLogging Global.vi" "Recording"(w382) -> ()
        n254 = property on="Camera Image" class="ImageControl"("Image Information Shown"=w374, "Image Information Visible"=w373) -> ()  [unwired: 2 in, 2 out]
        n255 = call <vilib>:"WPI_DashboardNT Log FieldName Cache.vi"("Operation"=enum16{"Lookup/Add", "Index", "Clear"}."Clear") -> ()  [unwired: 8 in, 3 out]
      }
      event Panel Close {
        w393 = enum32{"Stop", "Record", "Playback"}."Stop" ("Rec Mode")
        n256 = event-data() -> ()  [unwired: 1 in, 4 out]
        n257 = local write "Rec Mode"(w393) -> ()
        n258 = global write "WPI_DashboardLogging Global.vi" "Recording"(w393) -> ()
      }
      event Panel Close {
        # "Abort playback window and ourself"
        n259 = event-data() -> ()  [unwired: 1 in, 4 out]
        n260 = invoke class="VI" method="FP.Close"(reference=w398) -> (reference out=w397:refnum<vi>)  [unwired: 2 in, 2 out]
        n261 = invoke class="VI" method="Abort VI"(reference=w397) -> (error out=w396:errorcluster)  [unwired: 2 in, 2 out]
        n262 = invoke class="VI" method="Abort VI"(error in=w396) -> ()  [unwired: 2 in, 3 out]
      }
    }
  }
  n263 = property on="On/Off" class="Bool (strict)"("Visible"=w39) -> ()  [unwired: 2 in, 2 out]
  n264 = property on="Motor" class="Clust (strict)"("Visible"=w39) -> ()  [unwired: 2 in, 2 out]
  n265 = property on="Progress" class="Clust (strict)"("Visible"=w39) -> ()  [unwired: 2 in, 2 out]
  n266 = property on="Test Ring" class="Ring (strict)"("Visible"=w39) -> ()  [unwired: 2 in, 2 out]
  n267 = property on="Rev/Fwd" class="Clust (strict)"("Visible"=w39) -> ()  [unwired: 2 in, 2 out]
  n268 = property on="Camera Settings" class="Clust (strict)"("Visible"=w39) -> ()  [unwired: 2 in, 2 out]
  n269 = local write "DB Camera Config"(w39) -> ()
  n270 = global write "WPI_DashboardLogging Global.vi" "Recording"(w24) -> ()
  n271 = local write "Rec Mode"(w24) -> ()
  n272 = control-ref of="Autonomous\nMode"() -> (w1:refnum<vi>)
  n273 = call "DashboardSelectAuto.vi"("Table Prefix"="Autonomous mode", "Autonomous Mode Ring"=w1) -> ()  [unwired: 9 in]
